vi "launch nested actors.vi"(8 "error in (no error)":errorcluster, 11 "Template in":refnum<class "Template.lvclass">) -> (0 "error out":errorcluster, 3 "Template out":refnum<class "Template.lvclass">)   [LabVIEW 2020, in "Template.lvlib" / "Template.lvclass"]
uses:
  Template.lvclass
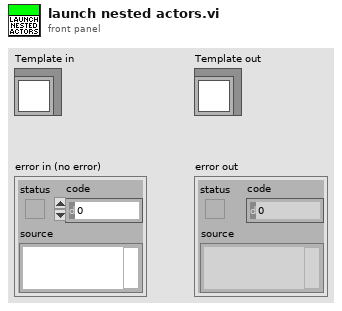
[diagram p1: front panel]
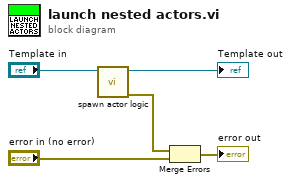
[diagram p0: block diagram]
diagram:
  n1 = call "spawn actor logic.vi"("Template in"="Template in") -> ("error out"=w1:errorcluster, "Template out"=→"Template out":refnum<class "Template.lvclass">)  [unwired: 9 in]
  n2 = Merge Errors(w1, "error in (no error)") -> (→"error out":errorcluster)
